vi "Manager UpdateClock.vi"(6 "contextId":T1, 8 "error in":errorcluster, 9 "timeout (ms)":i32=-1, 10 "Request Data":T3, 11 "gRPC ID":T1) -> (0 "error out":errorcluster, 2 "Response Data":T2, 3 "gRPC ID out":T1)   [LabVIEW 2021, in "CIF_Manager_client.lvlib"]
uses:
  CIF_Manager_client.lvlib
  <vilib>/gRPC/LabVIEW gRPC Library/Shared/grpcId.ctl
  RPC Messages/cif_manager_ClockUpdate.ctl
  RPC Messages/cif_manager_TimePair.ctl
  RPC Messages/cif_common_Status.ctl
  RPC Messages/cif_common_Status_Flat.ctl
  14035477-4c25-4107-8ed5-d0c4ef420ce5.vi
  RPC Messages/RichToFlatcif_manager_TimePair.vi
  <vilib>/gRPC/LabVIEW gRPC Library/Shared/TranslateGrpcError.vi
  <vilib>/gRPC/LabVIEW gRPC Library/Shared/Wait On Occurrence Wrapper.vi
  <vilib>/gRPC/LabVIEW gRPC Library/Shared/Wait On Occurence.vi
  <vilib>/gRPC/LabVIEW gRPC Library/Server API/Server/Get Server DLL Path.vi
  <vilib>/Utility/error.llb/Error Cluster From Error Code.vi
  <vilib>/Utility/config.llb/Open Config Data.vi
  <vilib>/Utility/config.llb/Write Key.vi
  <vilib>/Utility/config.llb/Write Key (Boolean).vi
  <vilib>/Utility/config.llb/Not A Config Data Refnum.vi
  <vilib>/Utility/config.llb/Read Key.vi
  <vilib>/Utility/config.llb/Read Key (Boolean).vi
  <vilib>/Utility/config.llb/Close Config Data.vi
  <vilib>/gRPC/LabVIEW gRPC Library/grpc-lvsupport-release.lvlib
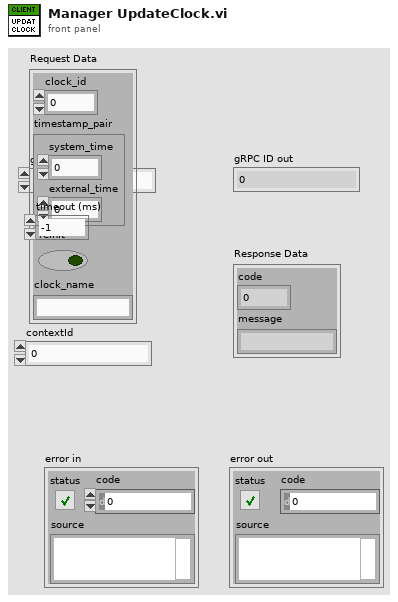
[diagram p1: front panel]
types:
  T1 = typedef "grpc-lvsupport-release.lvlib/grpcId.ctl" = u64
  T2 = typedef "CIF_Manager_client.lvlib/cif_common_Status.ctl" = cluster{"code":i32, "message":string}
  T3 = typedef "CIF_Manager_client.lvlib/cif_manager_ClockUpdate.ctl" = cluster{"clock_id":u32, "timestamp_pair":T4, "reinit":bool, "clock_name":string}
  T4 = typedef "CIF_Manager_client.lvlib/cif_manager_TimePair.ctl" = cluster{"system_time":i64, "external_time":i64}
  T5 = typedef "CIF_Manager_client.lvlib/cif_common_Status_Flat.ctl" = cluster{"code":i32, "message":string}
  T6 = typedef "CIF_Manager_client.lvlib/cif_manager_ClockUpdate_Flat.ctl" = cluster{"clock_id":u32, "timestamp_pair":T7, "reinit":bool, "clock_name":string}
  T7 = typedef "CIF_Manager_client.lvlib/cif_manager_TimePair_Flat.ctl" = cluster{"system_time":i64, "external_time":i64}
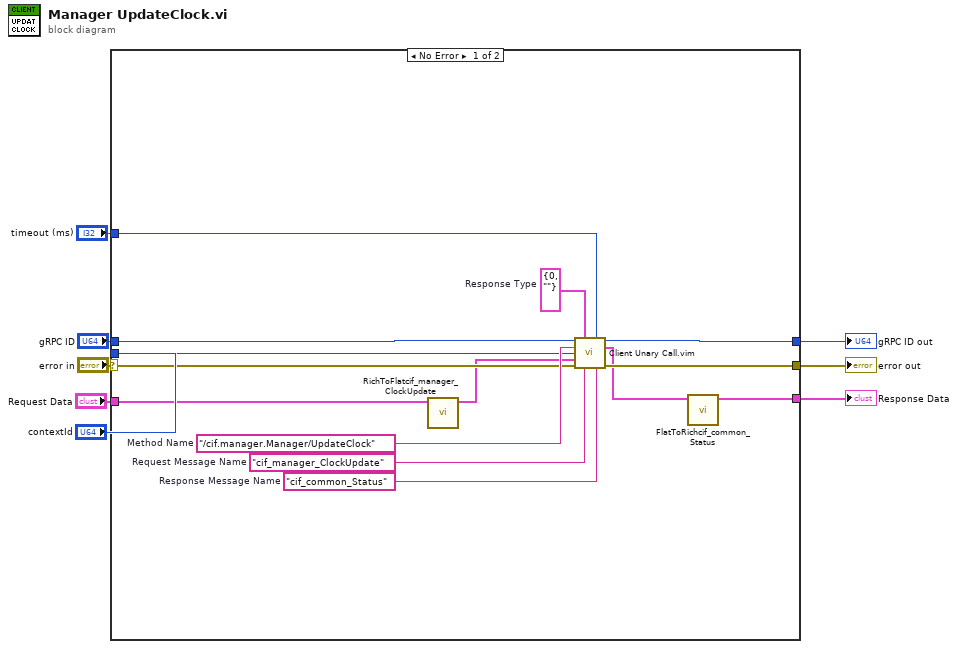
[diagram p0: block diagram]
diagram:
  n1 = case shown="No Error" "error in" {
    selector: "error in" -> [w18 w23]
    tunnel: [w17 w23] -> w7
    tunnel: "gRPC ID" -> [w16 w24]
    tunnel: [w15 w24] -> w5
    tunnel: "Request Data" -> [w12 _]
    tunnel: [w9 _] -> w3
    tunnel: "timeout (ms)" -> [w14 _]
    tunnel: "contextId" -> [w13 _]
    frame No Error {
      w19 = "cif_common_Status"  # Response Message Name
      w20 = "cif_manager_ClockUpdate"  # Request Message Name
      w21 = T5 {"code"=0, "message"=""}  # Response Type
      w22 = "/cif.manager.Manager/UpdateClock"  # Method Name
      n2 = call "RichToFlatcif_manager_ClockUpdate.vi"("InputCluster"=w12) -> ("OutputCluster"=w11:T6)  [unwired: 10 in]
      n3 = call "Client Unary Call.vim"("ClientID in"=w16, "Response Type"=w21, "timeout (ms)"=w14, "Method Name"=w22, "contextId"=w13, "Request Data"=w11, "error in"=w18, "Request Message Name"=w20, "Response Message Name"=w19) -> ("ClientID out"=w15:u64, "Response Data"=w10:T5, "error out"=w17:errorcluster)  [unwired: 4 in]
      n4 = call "FlatToRichcif_common_Status.vi"("InputCluster"=w10) -> ("OutputCluster"=w9:T2)  [unwired: 10 in]
    }
    frame Error {
    }
  }
  "error out" <- w7
  "gRPC ID out" <- w5
  "Response Data" <- w3
